vi "Configure Trigger Source.vi"(8 "error in (no error)":errorcluster, 10 "Source":string, 11 "Camera in":refnum<class "Camera.lvclass">) -> (0 "error out":errorcluster, 3 "Camera":refnum<class "Camera.lvclass">)   [LabVIEW 2020, in "Camera.lvclass"]
uses:
  Camera.lvclass
  Camera.lvclass/Camera.ctl
  bin/gindustrialcam_32-1.dll
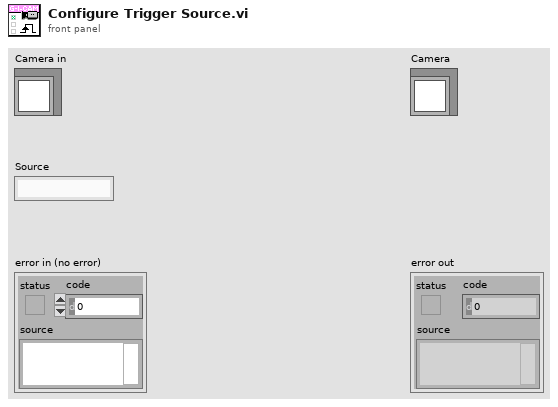
[diagram p1: front panel]
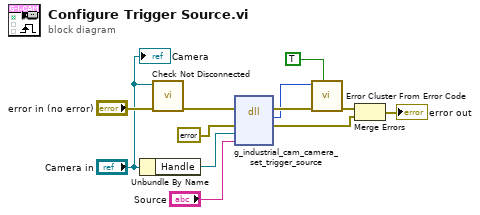
[diagram p0: block diagram]
diagram:
  n1 = Unbundle By Name("Camera in") -> ("Handle"=w4:refnum<data-value>)
  n2 = call "Check Not Disconnected.vi"("error in (no error)"="error in (no error)", "Camera in"="Camera in") -> ("error out"=w3:errorcluster)  [unwired: 9 in]
  n3 = dll-call lib="C:/Workspace/SSDC/g-industrial-camera/LabVIEW/g_industrial_cam/bin/gindustrialcam_*-1.*" fn="g_industrial_cam_camera_set_trigger_source"(error in=w3, "err"=errorcluster {"status"=FALSE, "code"=0, "source"=""} ("error constant"), "edvr"=w4, "source"="Source") -> (error out=w10:errorcluster, "Mg_Error"=w9:i32, "err"=w7:errorcluster)  [unwired: 4 in, 1 out]
  n4 = call <vilib>:"Error Cluster From Error Code.vi"("show call chain? (False)"=TRUE, "error in (no error)"=w10, "error code (0)"=w9) -> ("error out"=w8:errorcluster)  [unwired: 6 in]
  n5 = Merge Errors(w8, w7) -> (→"error out":errorcluster)
  "Camera" <- "Camera in"
